vi "Name_General Setup.vi"() -> (3 "Name":string)   [LabVIEW 2015, in "ConfigHelper.lvlib"]
uses:
  ConfigHelper.lvlib
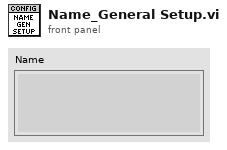
[diagram p1: front panel]
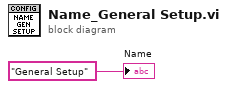
[diagram p0: block diagram]
diagram:
  "Name" <- "General Setup"
